vi "getBinaryValue.vi"(7 "Name":string, 8 "error in (no error)":errorcluster, 11 "tBSONDocument in":refnum<class "tBSONDocument.lvclass">) -> (0 "error out":errorcluster, 2 "Value":u8[](array[numeric]), 3 "tBSONDocument out":refnum<class "tBSONDocument.lvclass">)   [LabVIEW 2013, in "BSON.lvlib" / "tBSONDocument.lvclass"]
doc: "Retrieves a binary blob (an array of U8s) from a BSON document."
uses:
  tBSONDocument.lvclass
  BSONElements/tBSONBinary/tBSONBinary.lvclass
  BSONElements/tBSONBinary/getValue.vi
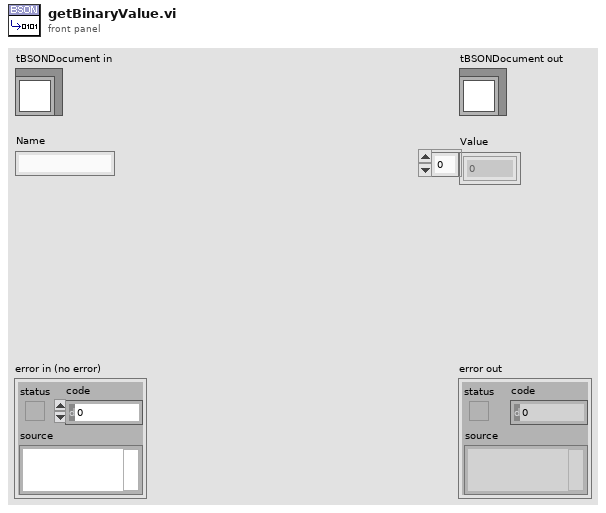
[diagram p1: front panel]
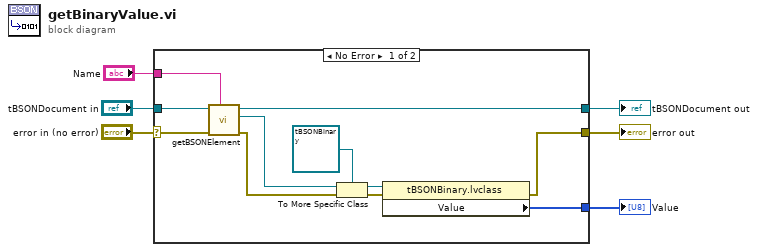
[diagram p0: block diagram]
diagram:
  n1 = case shown="No Error" "error in (no error)" {
    selector: "error in (no error)" -> [w9 w19]
    tunnel: [w8 w19] -> w5
    tunnel: [w7 w18] -> w3
    tunnel: "tBSONDocument in" -> [w17 w18]
    tunnel: "Name" -> [w16 _]
    tunnel: [w10 _] -> w1
    frame No Error {
      n2 = call "getBSONElement.vi"("Name"=w16, "error in (no error)"=w9, "tBSONDocument in"=w17) -> ("error out"=w15:errorcluster, "Element"=w14:refnum<class "tBSONElement.lvclass">, "tBSONDocument out"=w7:refnum<class "tBSONDocument.lvclass">)  [unwired: 6 in]
      n3 = To More Specific Class(target class=refnum<class "tBSONBinary.lvclass"> refnum ("lvMongoDriver.lvlib:BSON.lvlib:tBSONBinary.lvclass"), reference=w14, error in=w15) -> (specific class reference=w11:refnum<class "tBSONBinary.lvclass">, error out=w12:errorcluster)
      n4 = property class="tBSONBinary.lvclass"(reference=w11, error in=w12) -> (error out=w8:errorcluster, "Value"=w10:u8[])  [unwired: 1 out]
    }
    frame Error {
    }
  }
  "error out" <- w5
  "tBSONDocument out" <- w3
  "Value" <- w1
